vi "Get Handler by Name(by Ref).vi"(8 "error in (no error)":errorcluster, 10 "Handler Name":string) -> (0 "error out":errorcluster, 2 "Handler":refnum<class "Handler.lvclass">)   [LabVIEW 2017, in "Error Log.lvlib" / "Logger.lvclass"]
doc: "Returns the handler with the specified <b>Name</b> from the referenced ``*Logger``.\nIf name was not found, returns a basis handler without functionality and the error \"5030 - Item not found\" is returned."
uses:
  Logger.lvclass
  Handler/Handler.lvclass
  Logger.lvclass/Logger.ctl
  Get Handlers.vi
  Get Handler Names.vi
  <vilib>/Utility/error.llb/Error Cluster From Error Code.vi
  <vilib>/ErrorRing/Error Ring.xnode
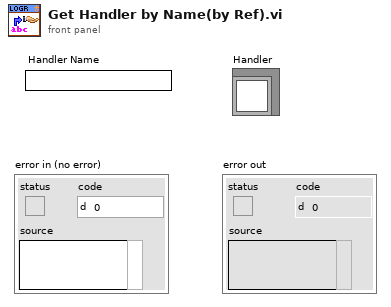
[diagram p1: front panel]
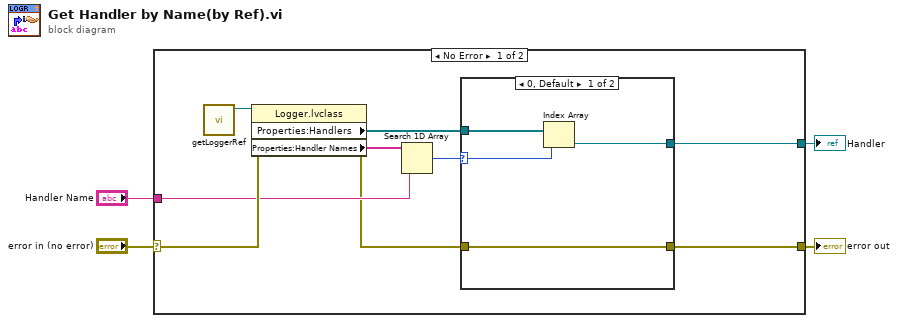
[diagram p0: block diagram]
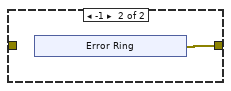
[diagram p2: hidden frame]
diagram:
  n1 = case shown="No Error" "error in (no error)" {
    selector: "error in (no error)" -> [w12 w24]
    tunnel: [w8 w24] -> w3
    tunnel: "Handler Name" -> [w11 _]
    tunnel: [w6 _] -> w1
    frame No Error {
      n2 = call "getLoggerRef.vi"() -> ("Logger Ref"=w5:refnum<data-value>)  [unwired: 10 in, 1 out]
      n3 = property class="Logger.lvclass"(reference=w5, error in=w12) -> (error out=w9:errorcluster, "Properties:Handlers"=w7:refnum<class "Handler.lvclass">[], "Properties:Handler Names"=w13:string[])  [unwired: 1 out]
      n4 = Search 1D Array(1D array=w13, element=w11) -> (index of element=w10:i32)  [unwired: 1 in]
      n5 = case shown="0, Default" w10 {
        selector: w10 -> [w16 _]
        tunnel: w9 -> [w14 _]
        tunnel: [w14 w18] -> w8
        tunnel: w7 -> [w17 _]
        tunnel: [w15 _] -> w6
        frame 0, Default {
          n6 = Index Array(array=w17, index=w16) -> (element=w15:refnum<class "Handler.lvclass">)
        }
        frame -1 {
          n7 = xnode "Error Ring"() -> ("error out"=w18:errorcluster)
        }
      }
    }
    frame Error {
    }
  }
  "error out" <- w3
  "Handler" <- w1
